vi "05 LV - Dataset Lifecycle.vi"() -> ()   [LabVIEW 2020]
uses:
  client/Dataset/Dataset.lvclass/Dataset.ctl
  client/Dataset/Dataset.lvclass
  client/Client/Client.lvclass
  client/DatasetCreateStaging/DatasetCreateStaging.lvclass
  client/List/List.lvclass
panel:
  out "created and found":bool
  out "rid":string
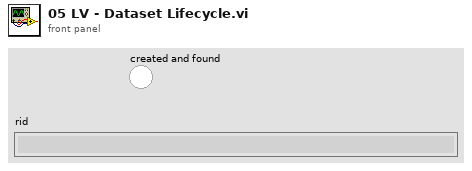
[diagram p1: front panel]
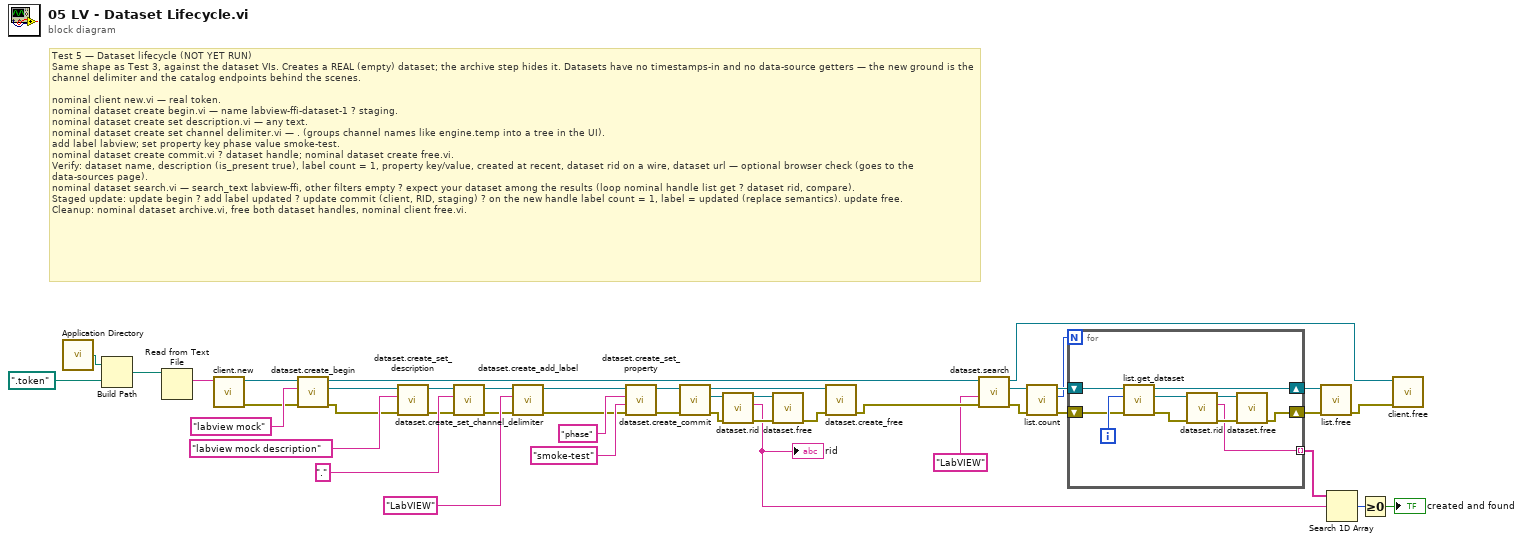
[diagram p0: block diagram]
diagram:
  # "Test 5 — Dataset lifecycle (NOT YET RUN)\nSame shape as Test 3, against the dataset VIs. Creates a REAL (empty) dataset; the archive step hides it. Datasets have no timestamps-in and no data-source getters — the new ground is the channel delimiter and the catalog endpoints behind the scenes.\n\nnominal client new.vi — real token.\nnominal dataset create begin.vi — name labview-ffi-dataset-1 ? staging.\nnominal dataset create set description.vi — any text.\nnominal dataset create set channel delimiter.vi — . (groups channel names like engine.temp into a tree in the UI).\nadd label labview; set property key phase value smoke-test.\nnominal dataset create commit.vi ? dataset handle; nominal dataset create free.vi.\nVerify: dataset name, description (is_present true), label count = 1, property key/value, created at recent, dataset rid on a wire, dataset url — optional browser check (goes to the data-sources page).\nnominal dataset search.vi — search_text labview-ffi, other filters empty ? expect your dataset among the results (loop nominal handle list get ? dataset rid, compare).\nStaged update: update begin ? add label updated ? update commit (client, RID, staging) ? on the new handle label count = 1, label = updated (replace semantics). update free.\nCleanup: nominal dataset archive.vi, free both dataset handles, nominal client free.vi."
  n1 = call <vilib>:"Application Directory.vi"() -> ("Application Directory"=w44:path)
  n2 = Build Path(base path=w44, name or relative path=path ".token") -> (appended path=w42:path)
  n3 = Read from Text File(file (use dialog)=w42) -> (text=w40:string)  [unwired: 3 in, 3 out]
  n4 = call "client.new.vi"("token"=w40) -> ("error out"=w39:errorcluster, "Client out"=w38:refnum<class "Client.lvclass">)  [unwired: 9 in]
  n5 = call "dataset.create_begin.vi"("error in"=w39, "name"="labview mock", "Client in"=w38) -> ("error out"=w35:errorcluster, "DatasetCreateStaging"=w36:refnum<class "DatasetCreateStaging.lvclass">, "Client out"=w16:refnum<class "Client.lvclass">)  [unwired: 6 in]
  n6 = call "dataset.create_set_description.vi"("error in"=w35, "description"="labview mock description" ("name"), "DatasetCreateStaging in"=w36) -> ("error out"=w32:errorcluster, "DatasetCreateStaging out"=w33:refnum<class "DatasetCreateStaging.lvclass">)  [unwired: 7 in]
  n7 = call "dataset.create_set_channel_delimiter.vi"("error in"=w32, "delimiter"="." ("name"), "DatasetCreateStaging in"=w33) -> ("error out"=w30:errorcluster, "DatasetCreateStaging out"=w29:refnum<class "DatasetCreateStaging.lvclass">)  [unwired: 7 in]
  n8 = call "dataset.create_add_label.vi"("error in"=w30, "label"="LabVIEW" ("name"), "DatasetCreateStaging in"=w29) -> ("error out"=w25:errorcluster, "DatasetCreateStaging out"=w26:refnum<class "DatasetCreateStaging.lvclass">)  [unwired: 7 in]
  n9 = call "dataset.create_set_property.vi"("error in"=w25, "value"="smoke-test" ("name"), "key"="phase" ("name"), "DatasetCreateStaging in"=w26) -> ("error out"=w23:errorcluster, "DatasetCreateStaging out"=w24:refnum<class "DatasetCreateStaging.lvclass">)  [unwired: 6 in]
  n10 = call "dataset.create_commit.vi"("error in"=w23, "DatasetCreateStaging in"=w24) -> ("error out"=w18:errorcluster, "Dataset"=w21:refnum<class "Dataset.lvclass">, "DatasetCreateStaging out"=w22:refnum<class "DatasetCreateStaging.lvclass">)  [unwired: 7 in]
  n11 = call "dataset.rid.vi"("error in"=w18, "Dataset in"=w21) -> ("error out"=w19:errorcluster, "rid"=w8:string, "Dataset out"=w20:refnum<class "Dataset.lvclass">)  [unwired: 7 in]
  "rid" <- w8
  n12 = call "dataset.free.vi"("error in"=w19, "Dataset"=w20) -> ("error out"=w17:errorcluster)  [unwired: 9 in]
  n13 = call "dataset.create_free.vi"("error in"=w17, "DatasetCreateStaging"=w22) -> ("error out"=w15:errorcluster)  [unwired: 9 in]
  n14 = call "dataset.search.vi"("error in"=w15, "label"="LabVIEW", "Client in"=w16) -> ("error out"=w4:errorcluster, "List"=w5:refnum<class "List.lvclass">, "Client out"=w11:refnum<class "Client.lvclass">)  [unwired: 6 in]
  n15 = call "list.count.vi"("error in"=w4, "List in"=w5) -> ("error out"=w3:errorcluster, "count"=w1:u32, "List out"=w2:refnum<class "List.lvclass">)  [unwired: 7 in]
  n16 = for {
    N: w1 -> [_]
    shift-right: [w52] -> w12
    shift-left: w3 -> [w45]
    shift-right: [w48] -> w13
    shift-left: w2 -> [w50]
    tunnel: [w51] -> w9 mode=indexing
    i -> [w49]
    n17 = call "list.get_dataset.vi"("error in (no error)"=w45, "index"=w49, "List in"=w50) -> ("error out"=w46:errorcluster, "Dataset"=w47:refnum<class "Dataset.lvclass">, "List out"=w48:refnum<class "List.lvclass">)  [unwired: 6 in]
    n18 = call "dataset.rid.vi"("error in"=w46, "Dataset in"=w47) -> ("error out"=w53:errorcluster, "rid"=w51:string, "Dataset out"=w54:refnum<class "Dataset.lvclass">)  [unwired: 7 in]
    n19 = call "dataset.free.vi"("error in"=w53, "Dataset"=w54) -> ("error out"=w52:errorcluster)  [unwired: 9 in]
  }
  n20 = call "list.free.vi"("error in"=w12, "List in"=w13) -> ("error out"=w10:errorcluster)  [unwired: 9 in]
  n21 = Search 1D Array(1D array=w9, element=w8) -> (index of element=w7:i32)  [unwired: 1 in]
  n22 = Greater Or Equal To 0?(x=w7) -> (x >= 0?=→"created and found":bool)
  n23 = call "client.free.vi"("error in"=w10, "Client in"=w11) -> ()  [unwired: 9 in, 1 out]
